vi "Write Config Settings to INI file.vi"(10 "Hardware Configuration":T1={"SEM X coil"="SEM-X", "SEM Y coil"="SEM-Y", "FIB X coil"="FIB/ao0", "FIB Y coil"="FIB/ao1", "FIB Detector"="FIB/ai1", "SEM Detectors"="Detectors", "Det min (V)"=-10.0, "Det max (V)"=10.0, "Eanable COM"=TRUE, "COM port"="COM1", "FIB Beam blank"="FIB/port0/line0", "FIB Ext Scan"="FIB/port0/line1", "Det. FIB-NI auto switch"="FIB/port0/line2", "Shutter Drive"="Log/ao0", "Machine Type"=2, "FIB Faraday Cup"="FIB/ai3", "Configuration file"=path "D:/3D FIB-SEM Files/Feiss.ini", "SEM Max FOV (um)"=350.0, "Machine ID"="Jeiss6/Merlin-xxxx", "Save config file"=FALSE, "Temperature port"="COM3", "Brightness A"=35.0, "Contrast A"=28.0, "Detector B name"="ESB @ 600 V", "Brightness B"=30.0, "Contrast B"=38.0, "Logging Device"="Log"} {"Machine Type" items=["Feiss", "NVision", "Jeiss"]}) -> ()   [LabVIEW 2018]
panel:
  out "String Lbls":string[](array[string])
  out "Numeric Lbls":string[](array[string])
  out "String Vals":string[](array[string])
  out "Numeric Vals":dbl[](array[numeric])
  out "Class Name":string[](array[string])
  out "Label text":string[](array[string])
  # "Detector"
  # "Brightness & Contrast (%)"
  # "A       InLens"
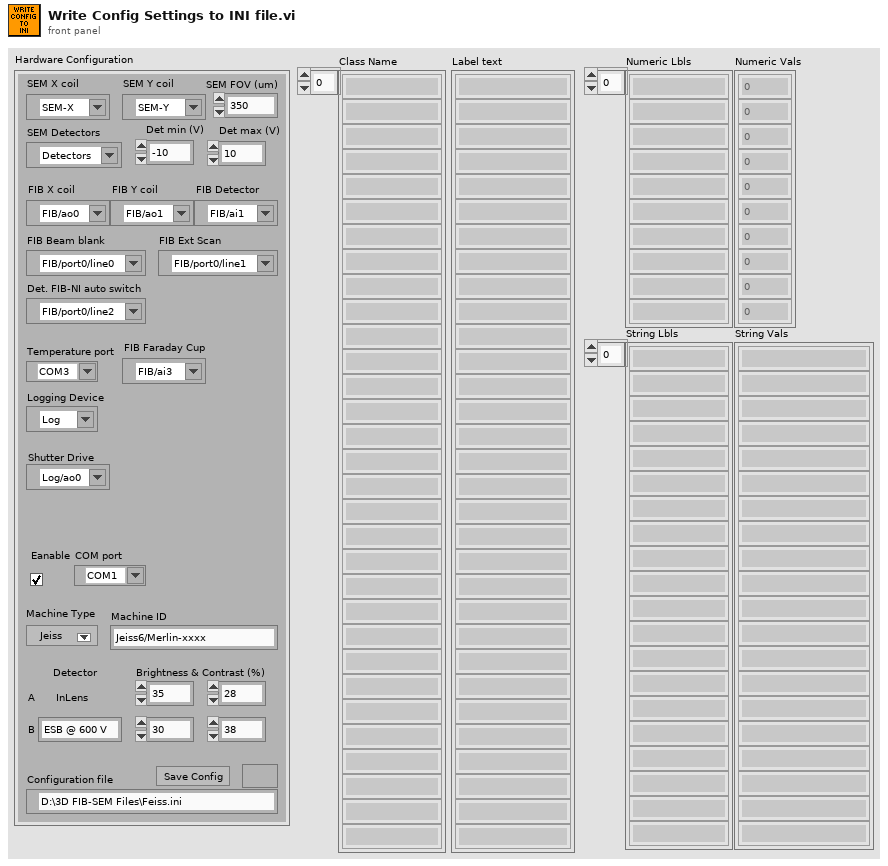
[diagram p1: front panel]
types:
  T1 = cluster{"SEM X coil":refnum<k15>, "SEM Y coil":refnum<k15>, "FIB X coil":tag, "FIB Y coil":tag, "FIB Detector":tag, "SEM Detectors":refnum<k15>, "Det min (V)":dbl, "Det max (V)":dbl, "Eanable COM":bool, "COM port":refnum<visa-resource-name>, "FIB Beam blank":tag, "FIB Ext Scan":tag, "Det. FIB-NI auto switch":tag, "Shutter Drive":tag, "Machine Type":u8, "FIB Faraday Cup":tag, "Configuration file":path, "SEM Max FOV (um)":sgl, "Machine ID":string, "Save config file":bool, "Temperature port":refnum<visa-resource-name>, "Brightness A":dbl, "Contrast A":dbl, "Detector B name":string, "Brightness B":dbl, "Contrast B":dbl, "Logging Device":tag}
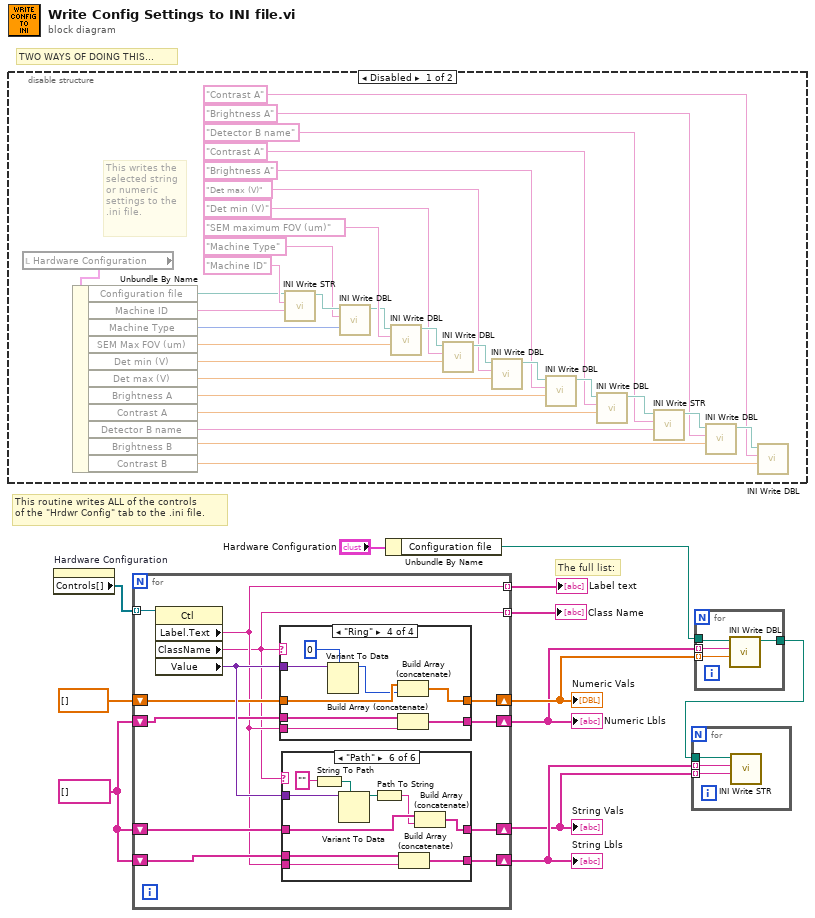
[diagram p0: block diagram]
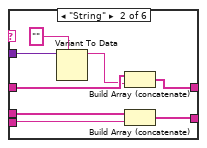
[diagram p4: hidden frame]
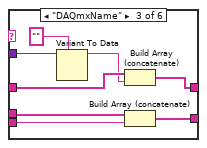
[diagram p5: hidden frame]
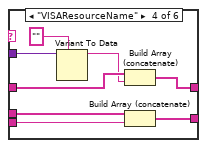
[diagram p6: hidden frame]
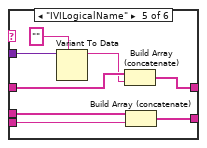
[diagram p7: hidden frame]
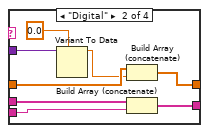
[diagram p9: hidden frame]
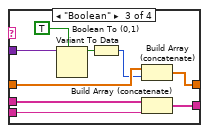
[diagram p10: hidden frame]
diagram:
  w3 = string[] []
  # "The full list:"
  # "TWO WAYS OF DOING THIS..."
  # "This routine writes ALL of the controls \nof the \"Hrdwr Config\" tab to the .ini file."
  n1 = disable-structure shown="Disabled" {
    frame Disabled {
      # "This writes the\nselected string \nor numeric \nsettings to the\n.ini file."
      n2 = local read "Hardware Configuration"() -> (w40:T1)
      n3 = Unbundle By Name(w40) -> ("Configuration file"=w41:path, "Machine ID"=w39:string, "Machine Type"=w35:u8, "SEM Max FOV (um)"=w33:sgl, "Det min (V)"=w32:dbl, "Det max (V)"=w27:dbl, "Brightness A"=w24:dbl, "Contrast A"=w22:dbl, "Detector B name"=w38:string, "Brightness B"=w18:dbl, "Contrast B"=w17:dbl)
      n4 = call "INI Write STR.vi"("Str Val In"=w39, "Key Str"="Machine ID", "configuration file path"=w41) -> ("file path Out"=w37:path)  [unwired: 7 in, 1 out]
      n5 = call "INI Write DBL.vi"("Value In"=w35, "Key Str"="Machine Type", "configuration file path"=w37) -> ("file path Out"=w34:path)  [unwired: 7 in, 1 out]
      n6 = call "INI Write DBL.vi"("Value In"=w33, "Key Str"="SEM maximum FOV (um)", "configuration file path"=w34) -> ("file path Out"=w31:path)  [unwired: 7 in, 1 out]
      n7 = call "INI Write DBL.vi"("Value In"=w32, "Key Str"="Det min (V)", "configuration file path"=w31) -> ("file path Out"=w29:path)  [unwired: 7 in, 1 out]
      n8 = call "INI Write DBL.vi"("Value In"=w27, "Key Str"="Det max (V)", "configuration file path"=w29) -> ("file path Out"=w25:path)  [unwired: 7 in, 1 out]
      n9 = call "INI Write DBL.vi"("Value In"=w24, "Key Str"="Brightness A", "configuration file path"=w25) -> ("file path Out"=w26:path)  [unwired: 7 in, 1 out]
      n10 = call "INI Write DBL.vi"("Value In"=w22, "Key Str"="Contrast A", "configuration file path"=w26) -> ("file path Out"=w20:path)  [unwired: 7 in, 1 out]
      n11 = call "INI Write STR.vi"("Str Val In"=w38, "Key Str"="Detector B name", "configuration file path"=w20) -> ("file path Out"=w16:path)  [unwired: 7 in, 1 out]
      n12 = call "INI Write DBL.vi"("Value In"=w18, "Key Str"="Brightness A", "configuration file path"=w16) -> ("file path Out"=w15:path)  [unwired: 7 in, 1 out]
      n13 = call "INI Write DBL.vi"("Value In"=w17, "Key Str"="Contrast A", "configuration file path"=w15) -> ()  [unwired: 7 in, 2 out]
    }
    frame Enabled {
    }
  }
  n14 = property on="Hardware Configuration" class="Clust (strict)"() -> ("Controls[]"=w12:refnum<vi>[])  [unwired: 2 in, 2 out]
  n15 = for {
    tunnel: w12 -> [w55] mode=indexing
    shift-right: [w52] -> w4
    shift-left: w3 -> [w53]
    shift-right: [w50] -> w8
    shift-left: dbl[] [] -> [w51]
    shift-right: [w48] -> w7
    shift-left: w3 -> [w49]
    shift-right: [w47] -> w5
    shift-left: w3 -> [w46]
    tunnel: [w45] -> w10 mode=indexing
    tunnel: [w44] -> w9 mode=indexing
    n16 = property class="Ctl"(reference=w55) -> ("Label.Text"=w45:string, "ClassName"=w44:string, "Value"=w54:variant)  [unwired: 1 in, 2 out]
    n17 = case shown="\"Ring\"" w44 {
      tunnel: w54 -> [_ w109 w118 w126]
      tunnel: w51 -> [w101 w107 w117 w125]
      tunnel: [w101 w105 w116 w124] -> w50
      tunnel: w45 -> [_ w102 w111 w122]
      tunnel: [w100 w104 w110 w121] -> w48
      tunnel: w49 -> [w100 w103 w112 w123]
      frame Default {
      }
      frame "Digital" {
        n18 = Variant To Data(type=0.0, Variant=w109) -> (data=w106:dbl)  [unwired: 1 in, 1 out]
        n19 = Build Array (concatenate)(w107, w106) -> (w105:dbl[])
        n20 = Build Array (concatenate)(w103, w102) -> (w104:string[])
      }
      frame "Boolean" {
        n21 = Variant To Data(type=TRUE, Variant=w118) -> (data=w114:bool)  [unwired: 1 in, 1 out]
        n22 = Boolean To (0,1)(Boolean=w114) -> (0, 1=w113:i16)
        n23 = Build Array (concatenate)(w117, w113) -> (w116:dbl[])
        n24 = Build Array (concatenate)(w112, w111) -> (w110:string[])
      }
      frame "Ring" {
        n25 = Variant To Data(type=u8 0, Variant=w126) -> (data=w119:u8)  [unwired: 1 in, 1 out]
        n26 = Build Array (concatenate)(w125, w119) -> (w124:dbl[])
        n27 = Build Array (concatenate)(w123, w122) -> (w121:string[])
      }
    }
    n28 = case shown="\"Path\"" w44 {
      tunnel: w54 -> [_ w65 w73 w81 w89 w94]
      tunnel: w53 -> [w57 w63 w71 w79 w87 w99]
      tunnel: [w57 w61 w69 w77 w85 w98] -> w52
      tunnel: w45 -> [_ w58 w66 w76 w84 w97]
      tunnel: [w56 w60 w68 w75 w83 w96] -> w47
      tunnel: w46 -> [w56 w59 w67 w74 w82 w95]
      frame Default {
      }
      frame "String" {
        n29 = Variant To Data(type="", Variant=w65) -> (data=w62:string)  [unwired: 1 in, 1 out]
        n30 = Build Array (concatenate)(w63, w62) -> (w61:string[])
        n31 = Build Array (concatenate)(w59, w58) -> (w60:string[])
      }
      frame "DAQmxName" {
        n32 = Variant To Data(type="", Variant=w73) -> (data=w70:string)  [unwired: 1 in, 1 out]
        n33 = Build Array (concatenate)(w71, w70) -> (w69:string[])
        n34 = Build Array (concatenate)(w67, w66) -> (w68:string[])
      }
      frame "VISAResourceName" {
        n35 = Variant To Data(type="", Variant=w81) -> (data=w78:string)  [unwired: 1 in, 1 out]
        n36 = Build Array (concatenate)(w79, w78) -> (w77:string[])
        n37 = Build Array (concatenate)(w74, w76) -> (w75:string[])
      }
      frame "IVILogicalName" {
        n38 = Variant To Data(type="", Variant=w89) -> (data=w86:string)  [unwired: 1 in, 1 out]
        n39 = Build Array (concatenate)(w87, w86) -> (w85:string[])
        n40 = Build Array (concatenate)(w82, w84) -> (w83:string[])
      }
      frame "Path" {
        n41 = String To Path(string="") -> (path=w93:path)
        n42 = Variant To Data(type=w93, Variant=w94) -> (data=w92:path)  [unwired: 1 in, 1 out]
        n43 = Path To String(path=w92) -> (string=w91:string)
        n44 = Build Array (concatenate)(w95, w97) -> (w96:string[])
        n45 = Build Array (concatenate)(w99, w91) -> (w98:string[])
      }
    }
  }
  "Label text" <- w10
  "Class Name" <- w9
  "Numeric Vals" <- w8
  "String Vals" <- w4
  "Numeric Lbls" <- w7
  "String Lbls" <- w5
  n46 = Unbundle By Name("Hardware Configuration") -> ("Configuration file"=w2:path)
  n47 = for {
    tunnel: w8 -> [w128] mode=indexing
    tunnel: w7 -> [w129] mode=indexing
    tunnel: w2 -> [w130]
    tunnel: [w127] -> w6
    n48 = call "INI Write DBL.vi"("Value In"=w128, "Key Str"=w129, "configuration file path"=w130) -> ("file path Out"=w127:path)  [unwired: 7 in, 1 out]
  }
  n49 = for {
    tunnel: w6 -> [w133]
    tunnel: w5 -> [w132] mode=indexing
    tunnel: w4 -> [w131] mode=indexing
    n50 = call "INI Write STR.vi"("Str Val In"=w131, "Key Str"=w132, "configuration file path"=w133) -> ()  [unwired: 7 in, 2 out]
  }
